vi "Processamento de imagem.vi"(0 "Image In":T2, 1 "Image Dst":T2, 2 "ROI Descriptor (Pattern Matching 1)":T1={"Global Rectangle"=[20, 20, 2284, 1516], "Contours"=[{"ID"=enum."External", "Type"=3, "Coordinates"=[20, 20, 2284, 1516]}]} {"Contours"."Type" items=["No Selection", "Point", "Line", "Rectangle", "Oval", "Polygon", "Freehand Region", "Annulus", "Unused2", "Unused3", "Broken Line", "Freehand Line", "Rotated Rectangle"]}, 5 "Template File Path":path=path "C:/Users/Acer/Documents/Tutiplast/Pino-Salcomp/template-pino.png", 7 "error in":errorcluster) -> (20 "Image Out":T2, 21 "Matches (Pattern Matching 1)":T3[](array[typedef]) {"Correlation Score" format="%.2f"; "Target Template Curve Score" format="%.2f"; "Template Target Curve Score" format="%.2f"; "Bounding Box"."y" format="%.2f"; "Bounding Box"."x" format="%.2f"; "Position"."y" format="%.2f"; "Position"."x" format="%.2f"; "Score" format="%.2f"; "Scale" format="%.2f"; "Angle" format="%.2f"; "Occlusion %" format="%.2f"}, 22 "Number of Matches (Pattern Matching 1)":i32, 27 "error out":errorcluster)   [LabVIEW 2020]
doc: "Creates, edits, and runs vision algorithms using NI Vision Assistant.\n\nWhen you place this Express VI on the block diagram, NI Vision Assistant launches. Create an algorithm using the Vision Assistant processing functions. After you create an algorithm, you can select the controls and indicators that you want to be able to programmatically set in LabVIEW. Double-click the Vision Assistant Express VI to edit the algorithm."
uses:
  <vilib>/vision/Image Controls.llb/IMAQ Image.ctl
  <vilib>/vision/Pattern Matching.llb/IMAQ GM Match Report.ctl
  <vilib>/vision/Pattern Matching.llb/IMAQ Curve Parameters.ctl
  <vilib>/vision/Pattern Matching.llb/IMAQ Match Range Setting.ctl
  <vilib>/vision/Pattern Matching.llb/IMAQ Geometric Pattern 2 Advanced Match Options.ctl
  <vilib>/vision/NI_Vision_Development_Module.lvlib
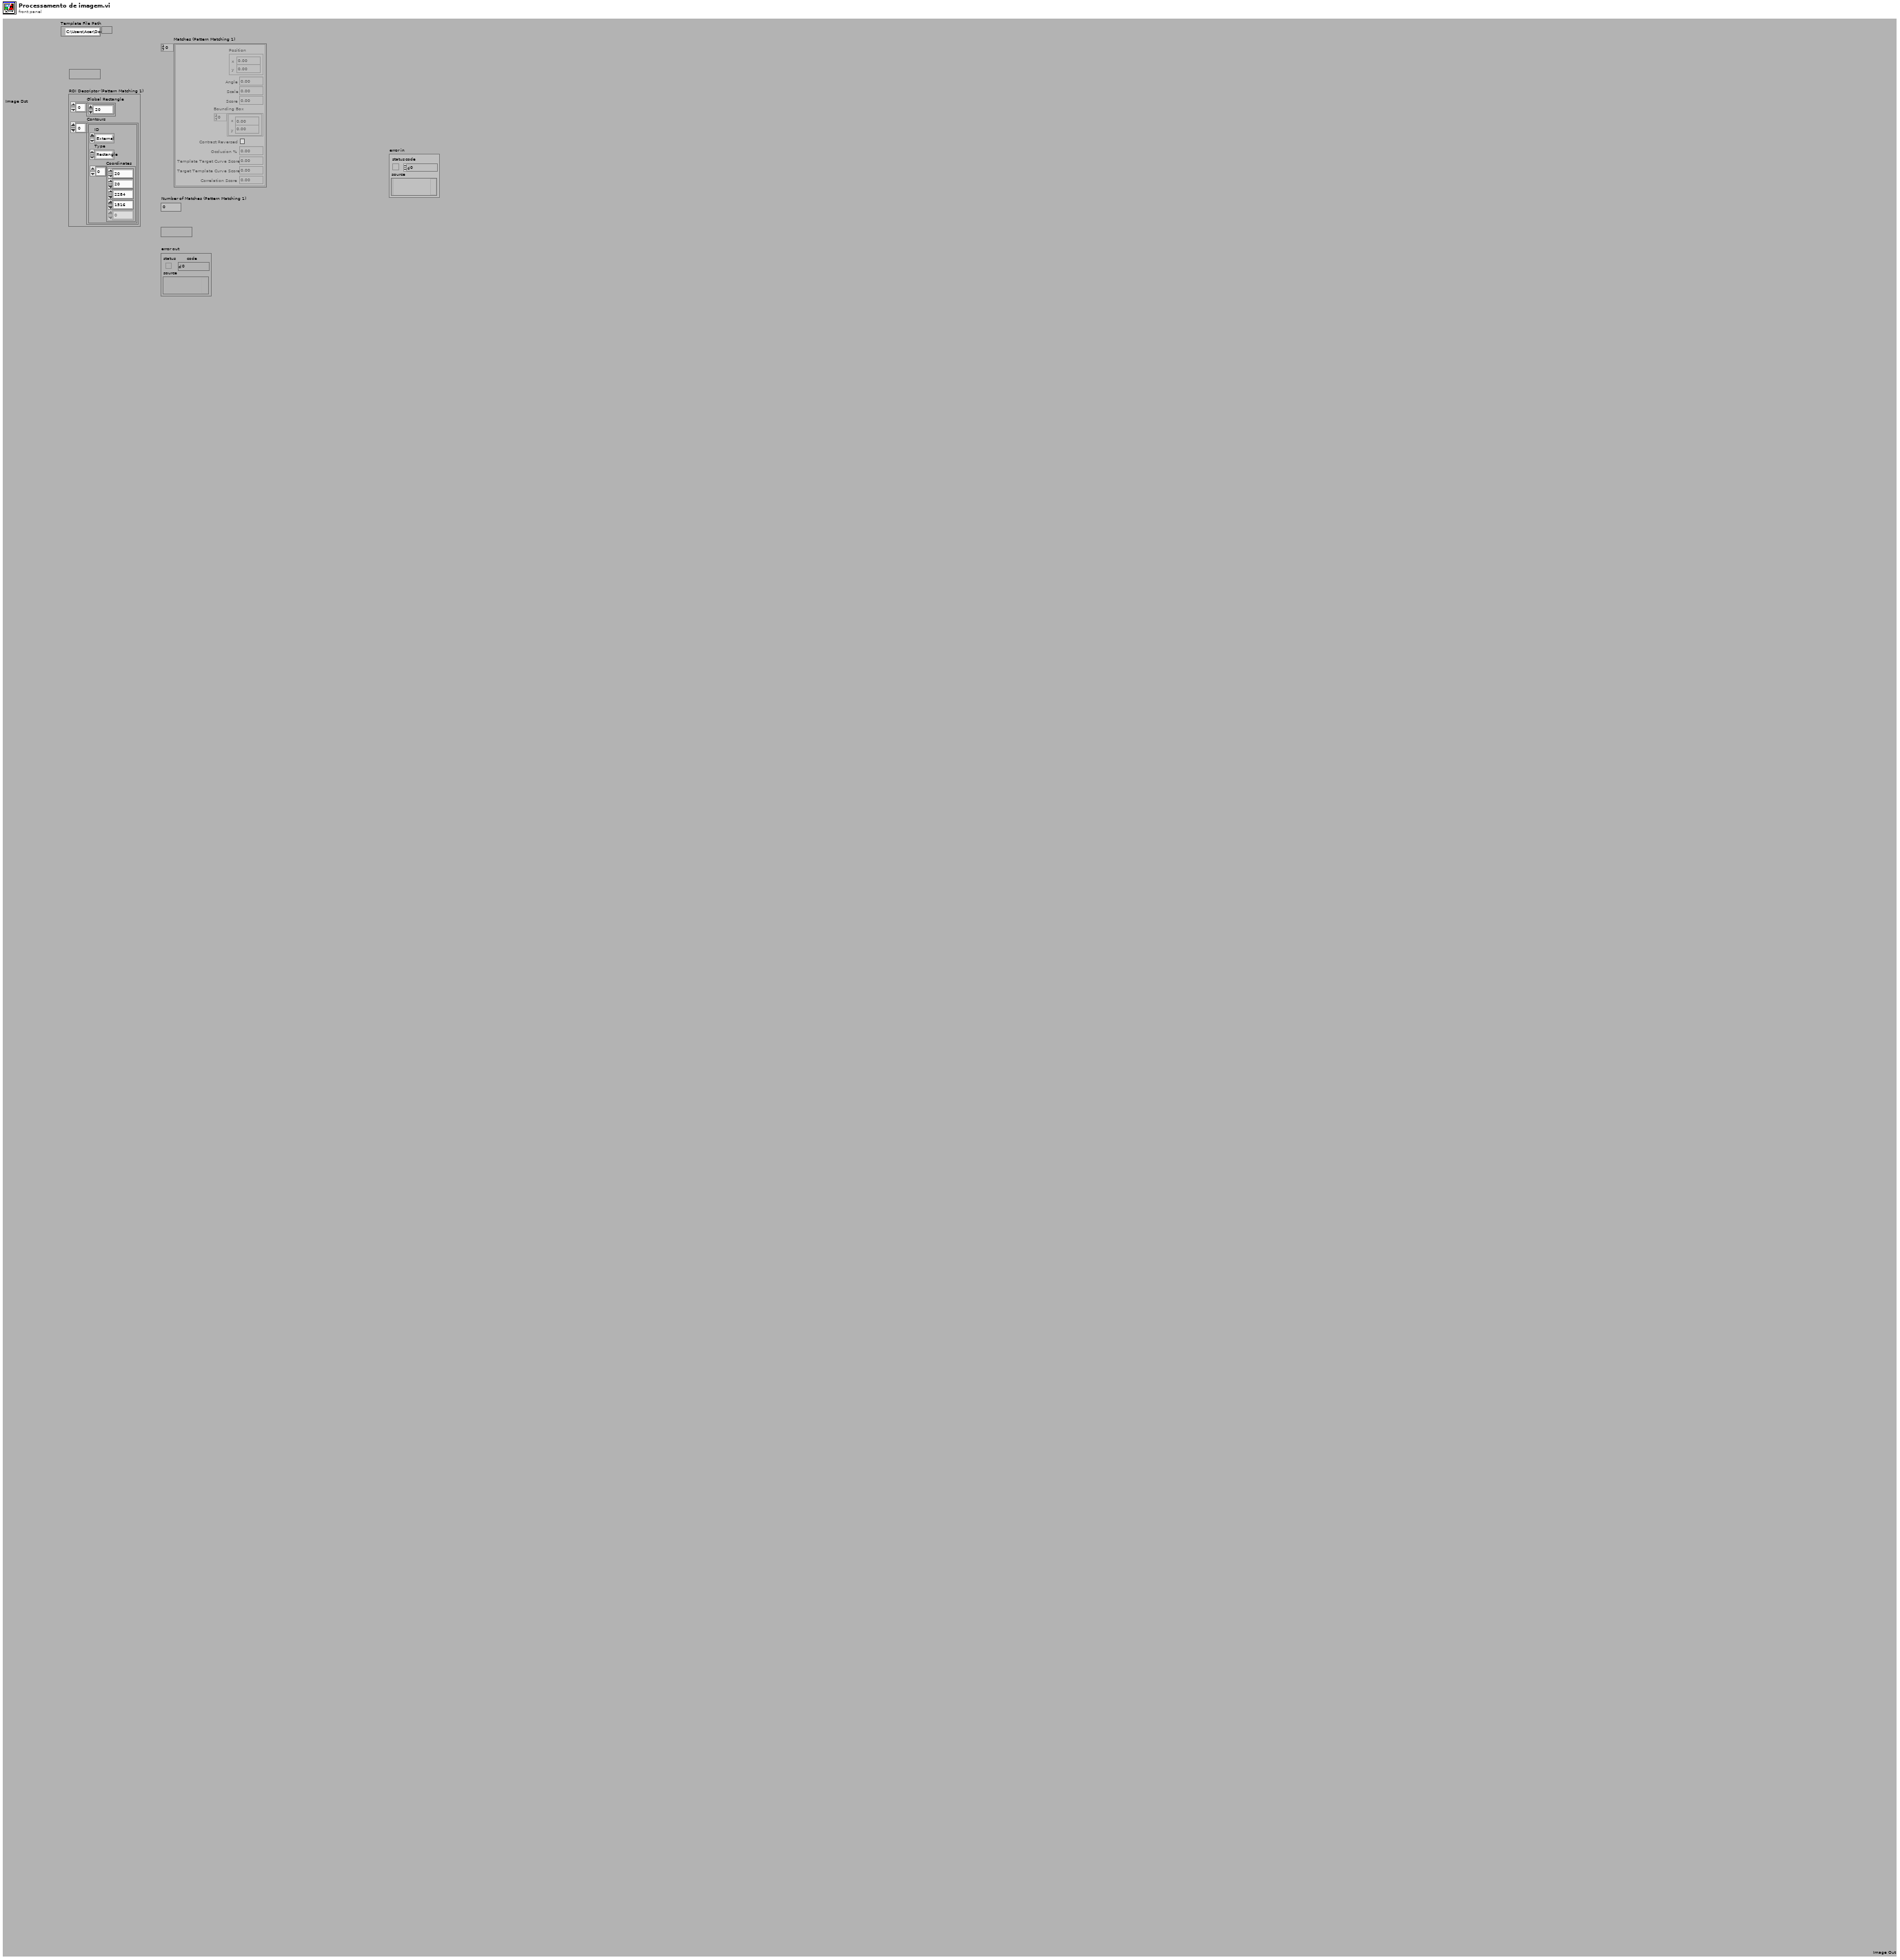
[diagram p1: front panel]
types:
  T1 = cluster{"Global Rectangle":i32[], "Contours":cluster{"ID":enum32{"External", "Internal"}, "Type":u32, "Coordinates":i32[]}[]}
  T2 = typedef "IMAQ Image.ctl" = refnum<image>
  T3 = typedef "IMAQ GM Match Report.ctl" = cluster{"Position":cluster{"x":sgl, "y":sgl}, "Angle":sgl, "Scale":sgl, "Score":sgl, "Bounding Box":cluster{"x":sgl, "y":sgl}[], "Contrast Reversed":bool, "Occlusion %":sgl, "Template Target Curve Score":sgl, "Target Template Curve Score":sgl, "Correlation Score":sgl}
  T4 = typedef "IMAQ Curve Parameters.ctl" = cluster{"Extraction Mode":u32, "Edge Threshold":i32, "Edge Filter Size":u32, "Min Length":i32, "Row Search Step Size":i32, "Col Search Step Size":i32, "Max Endpoint Gap":i32, "Closed":bool, "Subpixel":bool}
  T5 = typedef "IMAQ Match Range Setting.ctl" = cluster{"Match Constraints":u32, "Min":dbl, "Max":dbl}
  T6 = typedef "IMAQ Geometric Pattern 2 Advanced Match Options.ctl" = u16
  T7 = cluster{"Curve Parameters":T4, "Match Mode":cluster{"Rotation":bool, "Scale":bool, "Occlusion":bool, "Reserved 1":bool, "Reserved 2":bool, "Reserved 3":bool}, "Range Settings":T5[], "Number of Matches":i32, "Minimum Match Score":sgl, "SubPixel Accuracy":bool, "Adv. Geometric Match Options 2":cluster{"Setup Data Item":T6, "Item Value":dbl}[]}
  T8 = typedef "Image Type" = u32
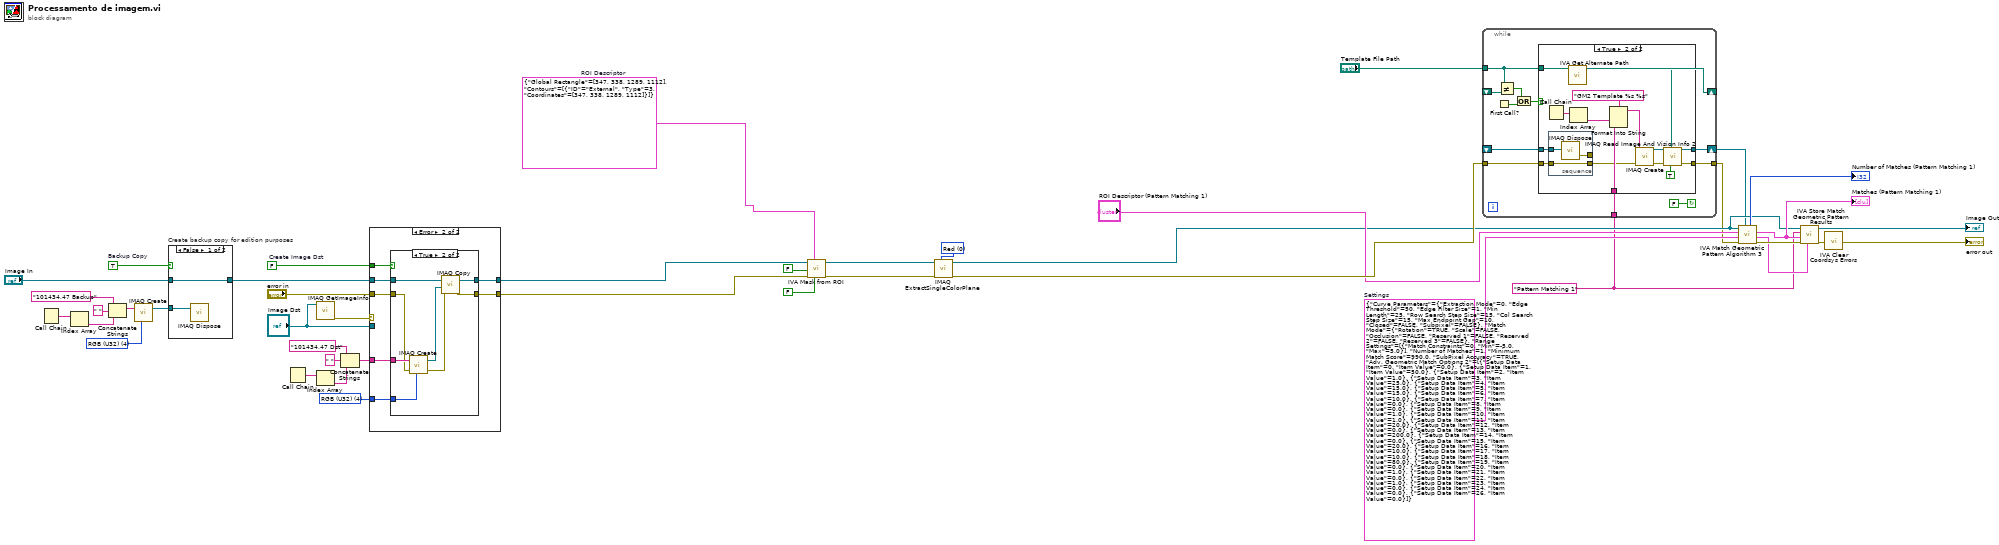
[diagram p0: block diagram]
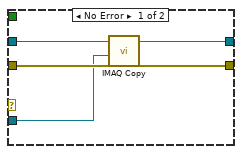
[diagram p3: hidden frame]
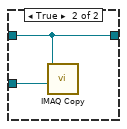
[diagram p5: hidden frame]
diagram:
  w7 = T7 {"Curve Parameters"={"Extraction Mode"=0, "Edge Threshold"=50, "Edge Filter Size"=1, "Min Length"=25, "Row Search Step Size"=15, "Col Search Step Size"=15, "Max Endpoint Gap"=10, "Closed"=FALSE, "Subpixel"=FALSE}, "Match Mode"={"Rotation"=TRUE, "Scale"=FALSE, "Occlusion"=FALSE, "Reserved 1"=FALSE, "Reserved 2"=FALSE, "Reserved 3"=FALSE}, "Range Settings"=[{"Match Constraints"=0, "Min"=-5.0, "Max"=5.0}], "Number of Matches"=1, "Minimum Match Score"=990.0, "SubPixel Accuracy"=TRUE, "Adv. Geometric Match Options 2"=[{"Setup Data Item"=0, "Item Value"=0.0}, {"Setup Data Item"=1, "Item Value"=50.0}, {"Setup Data Item"=2, "Item Value"=1.0}, {"Setup Data Item"=3, "Item Value"=25.0}, {"Setup Data Item"=4, "Item Value"=15.0}, {"Setup Data Item"=5, "Item Value"=15.0}, {"Setup Data Item"=6, "Item Value"=10.0}, {"Setup Data Item"=7, "Item Value"=0.0}, {"Setup Data Item"=8, "Item Value"=0.0}, {"Setup Data Item"=9, "Item Value"=1.0}, {"Setup Data Item"=10, "Item Value"=1.0}, {"Setup Data Item"=11, "Item Value"=20.0}, {"Setup Data Item"=12, "Item Value"=0.0}, {"Setup Data Item"=13, "Item Value"=200.0}, {"Setup Data Item"=14, "Item Value"=0.0}, {"Setup Data Item"=15, "Item Value"=20.0}, {"Setup Data Item"=16, "Item Value"=10.0}, {"Setup Data Item"=17, "Item Value"=10.0}, {"Setup Data Item"=18, "Item Value"=80.0}, {"Setup Data Item"=19, "Item Value"=0.0}, {"Setup Data Item"=20, "Item Value"=1.0}, {"Setup Data Item"=21, "Item Value"=0.0}, {"Setup Data Item"=22, "Item Value"=1.0}, {"Setup Data Item"=23, "Item Value"=0.0}, {"Setup Data Item"=24, "Item Value"=0.0}, {"Setup Data Item"=26, "Item Value"=0.0}]}  # Settings
  w6 = "Pattern Matching 1" ("Step Name")
  w17 = 0 items=["Red", "Green", "Blue", "Hue", "Saturation", "Luminance", "Value", "Intensity"] ("Color Plane")
  w22 = T1 {"Global Rectangle"=[347, 338, 1289, 1112], "Contours"=[{"ID"=enum."External", "Type"=3, "Coordinates"=[347, 338, 1289, 1112]}]}  # ROI Descriptor
  w23 = T8 4 items=["Grayscale (U8)", "Grayscale (I16)", "Grayscale (SGL)", "Complex (CSG)", "RGB (U32)", "HSL (U32)", "RGB (U64)", "Grayscale (U16)"] ("Image Dst Type")
  w24 = T8 4 items=["Grayscale (U8)", "Grayscale (I16)", "Grayscale (SGL)", "Complex (CSG)", "RGB (U32)", "HSL (U32)", "RGB (U64)", "Grayscale (U16)"] ("Image Type")
  w43 = TRUE  # Backup Copy
  w36 = FALSE  # Create Image Dst
  n1 = Call Chain() -> (call chain=w30:string[])
  n2 = Index Array(array=w30) -> (element=w29:string)  [unwired: 1 in]
  n3 = Concatenate Strings("101434,47 Backup" ("Backup Image Name"), " ", w29) -> (w26:string)
  n4 = call "IMAQ Create"("Image Name"=w26, "Image Type"=w24) -> ("New Image"=w25:T2)  [unwired: 2 in, 2 out]
  n5 = case "Create backup copy for edition purposes" shown="False" w43 {
    tunnel: [w45 w47] -> w39
    tunnel: "Image In" -> [w45 w47]
    tunnel: w25 -> [w44 w46]
    frame False {
      n6 = call "IMAQ Dispose"("Image"=w44) -> ()  [unwired: 2 in, 4 out]
    }
    frame True {
      n7 = call "IMAQ Copy"("Image Dst"=w46, "Image Src"=w47) -> ()  [unwired: 1 in, 5 out]
    }
  }
  n8 = Call Chain() -> (call chain=w35:string[])
  n9 = call "IMAQ GetImageInfo"("Image"="Image Dst") -> ("error out"=w41:errorcluster)  [unwired: 1 in, 9 out]
  n10 = Index Array(array=w35) -> (element=w33:string)  [unwired: 1 in]
  n11 = Concatenate Strings("101434,47 Dst" ("Image Dst Name"), " ", w33) -> (w31:string)
  n12 = case shown="Error" w41 {
    tunnel: [w52 w56] -> w20
    tunnel: [w51 w55] -> w37
    tunnel: w39 -> [w50 w57]
    tunnel: "error in" -> [w49 w53]
    tunnel: "Image Dst" -> [w48 _]
    tunnel: w31 -> [_ w59]
    tunnel: w23 -> [_ w58]
    tunnel: w36 -> [_ w54]
    frame No Error {
      n13 = call "IMAQ Copy"("error in (no error)"=w49, "Image Dst"=w48, "Image Src"=w50) -> ("error out"=w51:errorcluster, "Image Dst Out"=w52:T2)  [unwired: 3 out]
    }
    frame Error {
      n14 = case shown="True" w54 {
        tunnel: w59 -> [_ w69]
        tunnel: w58 -> [_ w68]
        tunnel: w57 -> [w61 w66]
        tunnel: [w61 w65] -> w56
        tunnel: [w60 w64] -> w55
        tunnel: w53 -> [w60 w62]
        frame False {
        }
        frame True {
          n15 = call "IMAQ Create"("Image Name"=w69, "Image Type"=w68, "error in (no error)"=w62) -> ("New Image"=w67:T2, "error out"=w63:errorcluster)  [unwired: 1 in, 1 out]
          n16 = call "IMAQ Copy"("error in (no error)"=w63, "Image Dst"=w67, "Image Src"=w66) -> ("error out"=w64:errorcluster, "Image Dst Out"=w65:T2)  [unwired: 3 out]
        }
      }
    }
  }
  n17 = call <vilib>:"IVA Mask from ROI.vi"("Shrink"=FALSE, "ROI Descriptor"=w22, "error in (no error)"=w37, "Out / In"=FALSE, "Image Src"=w20) -> ("error out"=w18:errorcluster, "Image Out"=w16:T2)  [unwired: 5 out]
  n18 = call "IMAQ ExtractSingleColorPlane"("Color Plane"=w17, "error in (no error)"=w18, "Image Src"=w16) -> ("error out"=w15:errorcluster, "Image Dst Out"=w8:T2)  [unwired: 1 in, 6 out]
  n19 = while {
    shift-right: [w80] -> w4
    shift-left: _ -> [w79]
    tunnel: [w77] -> w5
    tunnel: w15 -> [w76]
    tunnel: "Template File Path" -> [w73]
    tunnel: w6 -> [w75]
    shift-right: [w73] -> _
    shift-left: _ -> [w74]
    stop <- FALSE continue-if-true
    n20 = First Call?() -> (First Call?: T/F=w72:bool)
    n21 = Not Equal?(x=w73, y=w74) -> (x != y?=w71:bool)
    n22 = Or(x=w71, y=w72) -> (x .or. y?=w70:bool)
    n23 = case shown="True" w70 {
      tunnel: [w82 w84] -> w80
      tunnel: w79 -> [w82 w91]
      tunnel: [w81 w86] -> w77
      tunnel: w76 -> [w81 w92]
      tunnel: w75 -> [_ w93]
      tunnel: w73 -> [_ w90]
      frame False {
      }
      frame True {
        n24 = Call Chain() -> (call chain=w95:string[])
        n25 = stacked-sequence {
          tunnel: w92 -> [w100]
          tunnel: w91 -> [w99]
          tunnel: [w100] -> w89
          tunnel: [w98] -> _
          frame #0 {
            n26 = call "IMAQ Dispose"("Image"=w99) -> ("error out"=w98:errorcluster)  [unwired: 2 in, 3 out]
          }
        }
        n27 = call <vilib>:"IVA Get Alternate Path.vi"("Path In"=w90) -> ("Path Out"=w85:path)  [unwired: 10 out]
        n28 = Index Array(array=w95) -> (element=w94:string)  [unwired: 1 in]
        n29 = Format Into String(format string="GM2 Template %s %s" ("Image Name"), w94, w93) -> (resulting string=w97:string)  [unwired: 2 in, 1 out]
        n30 = call "IMAQ Create"("Image Name"=w97, "error in (no error)"=w89) -> ("New Image"=w83:T2, "error out"=w87:errorcluster)  [unwired: 2 in, 1 out]
        n31 = call "IMAQ Read Image And Vision Info 2"("Use File Path Image Type"=TRUE, "File Path"=w85, "error in (no error)"=w87, "Image"=w83) -> ("error out"=w86:errorcluster, "Image Out"=w84:T2)  [unwired: 5 in, 1 out]
      }
    }
  }
  n32 = call <vilib>:"IVA Match Geometric Pattern Algorithm 3.vi"("Template"=w4, "error in (no error)"=w5, "Settings"=w7, "ROI Descriptor"="ROI Descriptor (Pattern Matching 1)", "Image"=w8) -> ("error out"=w12:errorcluster, "Calibrated Matches"=w10:T3[], "Matches"=w11:T3[], "Number of Matches"=→"Number of Matches (Pattern Matching 1)":i32)  [unwired: 3 out]
  "Matches (Pattern Matching 1)" <- w11
  n33 = call <vilib>:"IVA Store Match Geometric Pattern Results.vi"("Calibrated Matches"=w10, "error in (no error)"=w12, "Matches"=w11, "Step Name"=w6, "Image in"=w8) -> ("error out"=w3:errorcluster, "Image dup"=→"Image Out":T2)  [unwired: 5 out]
  n34 = call <vilib>:"IVA Clear Coordsys Errors.vi"("error in (no error)"=w3) -> ("error out"=→"error out":errorcluster)  [unwired: 10 in]
